vi "Handle Tree Run Time Menu Item Select.vi"(6 "Coords":T1, 8 "error in (no error)":errorcluster, 9 "ItemPath":string, 10 "ItemTag":string, 11 "File Explorer in":refnum<class "File Explorer.lvclass">) -> (0 "error out":errorcluster, 3 "File Explorer out":refnum<class "File Explorer.lvclass">)   [LabVIEW 2019, in "File Explorer.lvlib" / "File Explorer.lvclass"]
doc: "<RequiredOverrideReason>The action to take for a given Right-click run time menu selection in the file explorer tree.</RequiredOverrideReason>"
uses:
  <vilib>/gpm_packages/@cs/file-explorer-extension/Source/File Explorer/File Explorer/File Explorer.lvclass
  <vilib>/Utility/miscctls.llb/LVPoint32TypeDef.ctl
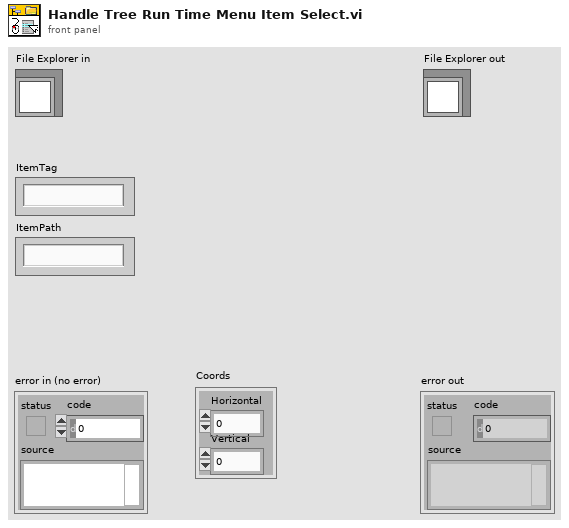
[diagram p1: front panel]
types:
  T1 = typedef "LVPoint32TypeDef.ctl" = cluster{"Horizontal":i32, "Vertical":i32}
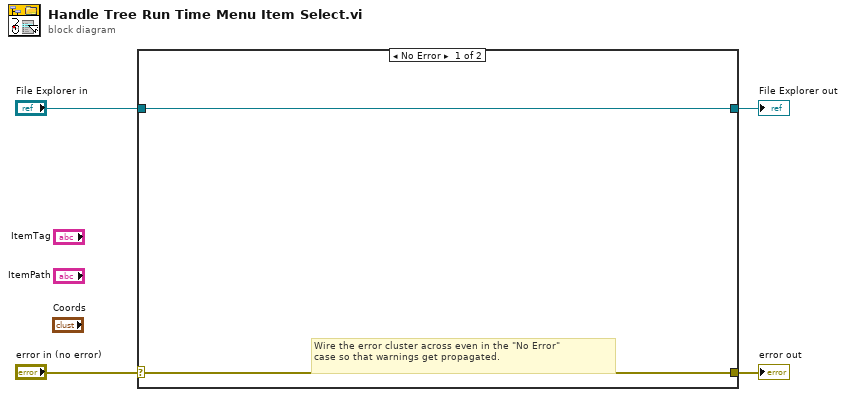
[diagram p0: block diagram]
diagram:
  n1 = case shown="No Error" "error in (no error)" {
    selector: "error in (no error)" -> [w5 w8]
    tunnel: [w5 w8] -> w3
    tunnel: [w6 w7] -> w1
    tunnel: "File Explorer in" -> [w6 w7]
    frame No Error {
      # "Wire the error cluster across even in the \"No Error\"\ncase so that warnings get propagated."
    }
    frame Error {
    }
  }
  "error out" <- w3
  "File Explorer out" <- w1
